vi "Create Error Trace.vi"(7 "Trace Source":string, 9 "Error In":errorcluster, 10 "Instance Name":string, 11 "System Name":string) -> (2 "Trace":refnum<class "Trace.lvclass">)   [LabVIEW 2014, in "Robot Actor Framework.lvlib" / "Trace.lvlib" / "Trace.lvclass"]
uses:
  Trace.lvclass
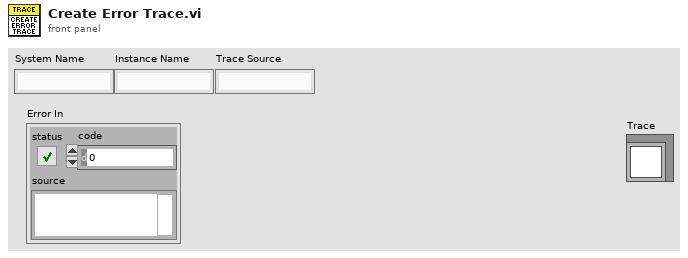
[diagram p1: front panel]
types:
  T1 = enum16{"Critical", "Error", "Warning", "Informational", "Debug"}
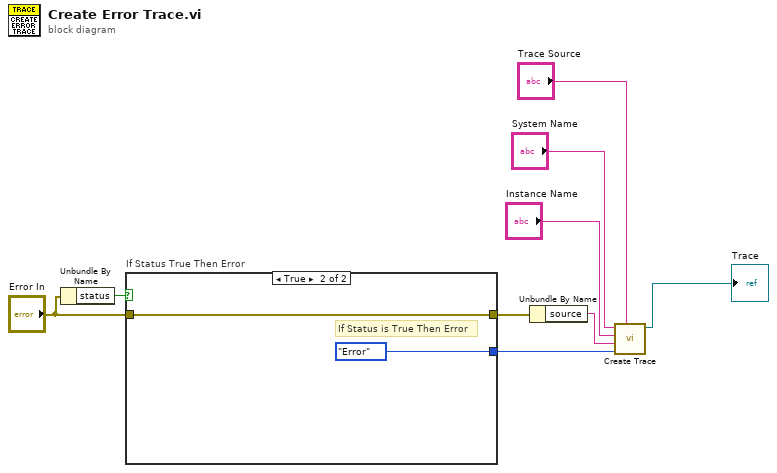
[diagram p0: block diagram]
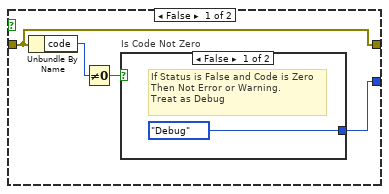
[diagram p2: hidden frame]
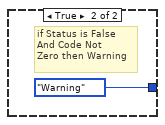
[diagram p3: hidden frame]
diagram:
  n1 = Unbundle By Name("Error In") -> ("status"=w9:bool)
  n2 = case "If Status True Then Error" shown="True" w9 {
    tunnel: [w12 T1."Error" ("Trace Level")] -> w6
    tunnel: "Error In" -> [w11 w16]
    tunnel: [w11 w16] -> w7
    frame False {
      n3 = Unbundle By Name(w11) -> ("code"=w10:i32)
      n4 = Not Equal To 0?(x=w10) -> (x != 0?=w13:bool)
      n5 = case "Is Code Not Zero" shown="False" w13 {
        tunnel: [T1."Debug" ("Trace Level") T1."Warning" ("Trace Level")] -> w12
        frame False {
          # "If Status is False and Code is Zero\nThen Not Error or Warning.\nTreat as Debug"
        }
        frame True {
          # "if Status is False\nAnd Code Not\nZero then Warning"
        }
      }
    }
    frame True {
      # "If Status is True Then Error"
    }
  }
  n6 = Unbundle By Name(w7) -> ("source"=w3:string)
  n7 = call "Create Trace.vi"("Trace Source"="Trace Source", "Trace Level"=w6, "Trace Message"=w3, "Instance Name"="Instance Name", "System Name"="System Name") -> ("Trace"=→"Trace":refnum<class "Trace.lvclass">)  [unwired: 6 in]
